vi "ReadyState.vi"(8 "error in (no error)":errorcluster, 10 "Cluster in":T2, 11 "Enum in":T1) -> (0 "error out":errorcluster, 2 "Cluster out":T2, 3 "Enum":T1)   [LabVIEW 2018]
uses:
  Type_Def/Type_Def Actuator Controls.ctl
  Type_Def/Type_Def ControlState.ctl
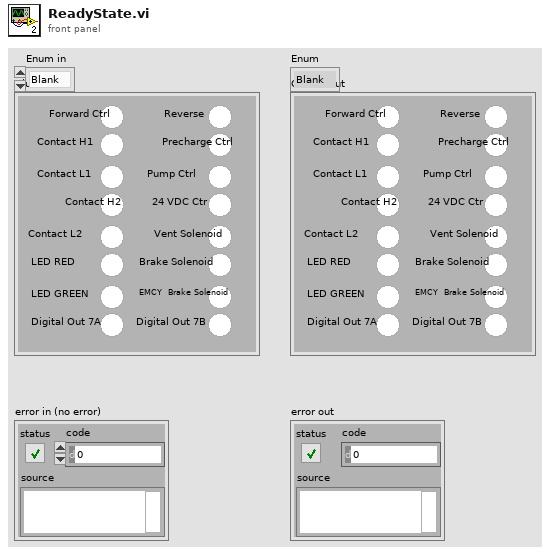
[diagram p1: front panel]
types:
  T1 = typedef "Type_Def ControlState.ctl" = enum16{"Blank", "Systems Check", "Idle", "Ready", "Pushing", "CrawlingPrecharge", "Braking", "Fault", "Boot Up", "Unpowered", "Crawling", "Shutdown", "Service Push", "Service Wait", "Vent", "Precharge"}
  T2 = typedef "Type_Def Actuator Controls.ctl" = cluster{"Reverse ":bool, "Precharge Ctrl":bool, "Pump Ctrl":bool, "24 VDC Ctr":bool, "Vent Solenoid":bool, "Brake Solenoid":bool, "EMCY  Brake Solenoid":bool, "Digital Out 7B ":bool, "Forward Ctrl":bool, "Contact H1":bool, "Contact L1":bool, "Contact H2":bool, "Contact L2 ":bool, "LED RED":bool, "LED GREEN":bool, " Digital Out 7A":bool}
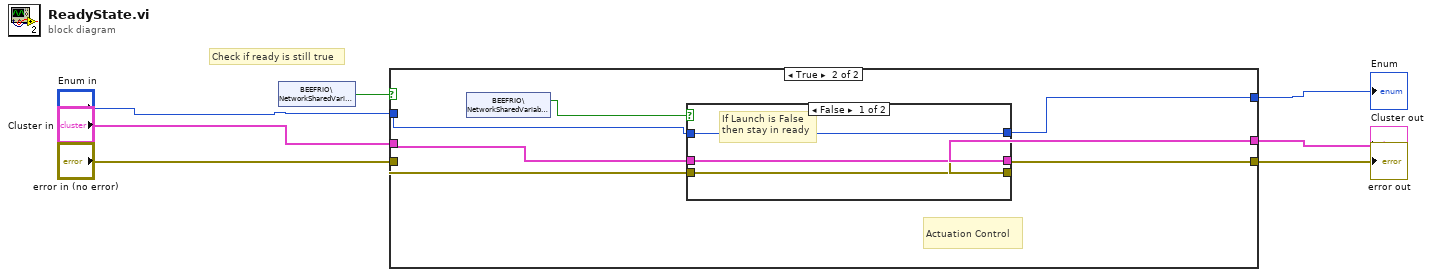
[diagram p0: block diagram]
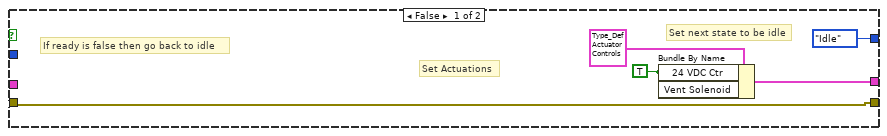
[diagram p2: hidden frame]
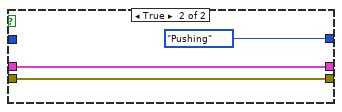
[diagram p3: hidden frame]
diagram:
  # "Check if ready is still true"
  n1 = shared-variable "BEEFRIO\\NetworkSharedVariable.lvlib\\Ready"() -> (w7:bool)  [unwired: 1 in, 1 out]
  n2 = case shown="True" w7 {
    tunnel: "Enum in" -> [_ w19]
    tunnel: [Type_Def_ControlState."Idle" w18] -> w2
    tunnel: "Cluster in" -> [_ w17]
    tunnel: [w9 w16] -> w4
    tunnel: [w8 w15] -> w5
    tunnel: "error in (no error)" -> [w8 w14]
    frame False {
      w11 = TRUE
      # "Set next state to be idle"
      # "Set Actuations"
      # "If ready is false then go back to idle"
      n3 = Bundle By Name(cluster=T2 {"Reverse "=FALSE, "Precharge Ctrl"=FALSE, "Pump Ctrl"=FALSE, "24 VDC Ctr"=FALSE, "Vent Solenoid"=FALSE, "Brake Solenoid"=FALSE, "EMCY  Brake Solenoid"=FALSE, "Digital Out 7B "=FALSE, "Forward Ctrl"=FALSE, "Contact H1"=FALSE, "Contact L1"=FALSE, "Contact H2"=FALSE, "Contact L2 "=FALSE, "LED RED"=FALSE, "LED GREEN"=FALSE, " Digital Out 7A"=FALSE}, "24 VDC Ctr"=w11, "Vent Solenoid"=w11) -> (w9:T2)
    }
    frame True {
      # "Actuation Control"
      n4 = shared-variable "BEEFRIO\\NetworkSharedVariable.lvlib\\Launch"() -> (w13:bool)  [unwired: 1 in, 1 out]
      n5 = case shown="False" w13 {
        tunnel: w19 -> [w21 _]
        tunnel: [w21 Type_Def_ControlState."Pushing"] -> w18
        tunnel: w17 -> [w20 w23]
        tunnel: [w20 w23] -> w16
        tunnel: [w22 w24] -> w15
        tunnel: w14 -> [w22 w24]
        frame False {
          # "If Launch is False \nthen stay in ready"
        }
        frame True {
        }
      }
    }
  }
  "error out" <- w5
  "Cluster out" <- w4
  "Enum" <- w2
